vi "Intensity integral - Copy.vi"(1 "width":i32, 2 "begin":i32, 3 "数组":dbl[][](array[numeric])) -> (0 "数组 2":dbl[](array[numeric]))   [LabVIEW 2018]
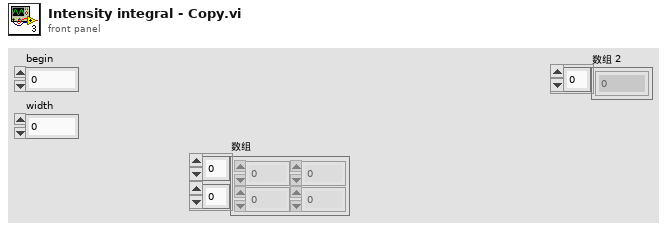
[diagram p1: front panel]
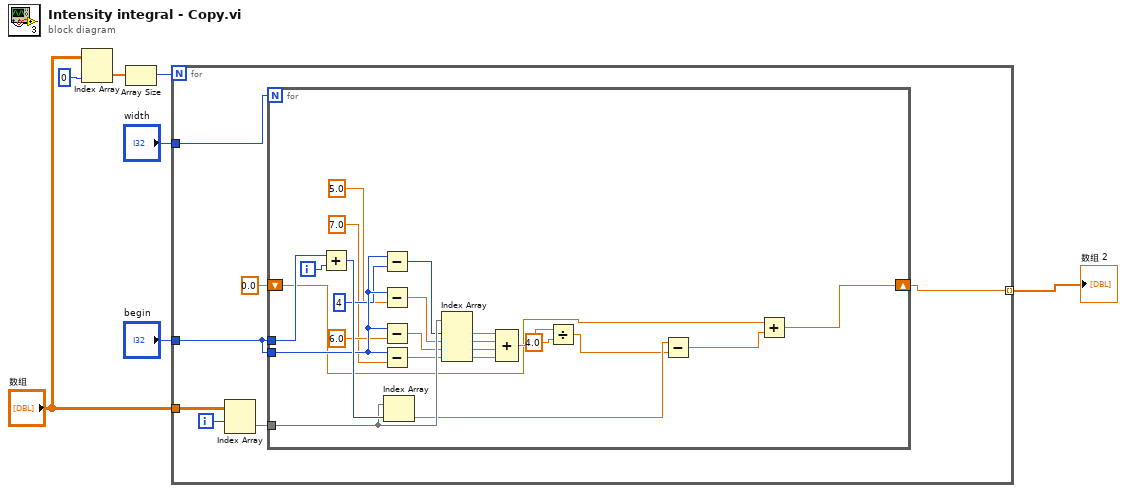
[diagram p0: block diagram]
diagram:
  n1 = Index Array(array="数组", index (col)=0 ("禁用的索引 (列)")) -> (element=w5:dbl[])  [unwired: 1 in]
  n2 = Array Size(array=w5) -> (size(s)=w2:i32)
  n3 = for {
    N: w2 -> [_]
    tunnel: "数组" -> [w14]
    tunnel: "begin" -> [w10]
    tunnel: "width" -> [w11]
    tunnel: [w8] -> w1 mode=indexing
    i -> [w13]
    n4 = Index Array(array=w14, index (row)=w13) -> (element=w12:dbl[])  [unwired: 1 in]
    n5 = for {
      N: w11 -> [_]
      tunnel: w12 -> [w35]
      tunnel: w10 -> [w37]
      tunnel: w10 -> [w30]
      shift-right: [w16] -> w8
      shift-left: 0.0 -> [w15]
      i -> [w38]
      n6 = Add(x=w37, y=w38) -> (x+y=w36:i32)
      n7 = Subtract(x=w30, y=4) -> (x-y=w34:i32)
      n8 = Subtract(x=w30, y=5.0) -> (x-y=w33:dbl)
      n9 = Subtract(x=w30, y=6.0) -> (x-y=w32:dbl)
      n10 = Subtract(x=w30, y=7.0) -> (x-y=w31:dbl)
      n11 = Index Array(array=w35, index=w36) -> (element=w19:dbl)
      n12 = Index Array(array=w35, index #1=w34, index #2=w33, index #3=w32, index #4=w31) -> (element #1=w25:dbl, element #2=w24:dbl, element #3=w23:dbl, element #4=w22:dbl)
      n13 = Compound Arithmetic op=unknown(w25, w24, w23, w22) -> (w21:dbl)
      n14 = Divide(x=w21, y=4.0) -> (x/y=w18:dbl)
      n15 = Subtract(x=w19, y=w18) -> (x-y=w17:dbl)
      n16 = Add(x=w15, y=w17) -> (x+y=w16:dbl)
    }
  }
  "数组 2" <- w1
